vi "write wav file.vi"() -> ()   [LabVIEW 2018]
panel:
  in  "#Channels":i32=1
  in  "Device":u32
  in  "Resolution (bits)":i32=16
  in  "Sample rate (Hz)":dbl=44100.0
  in  "Path for Audio 1":path
  out "path out for Audio 1":path
  in  "Path for Audio 2":path
  out "Waveform Graph":dynamicdata(graph)
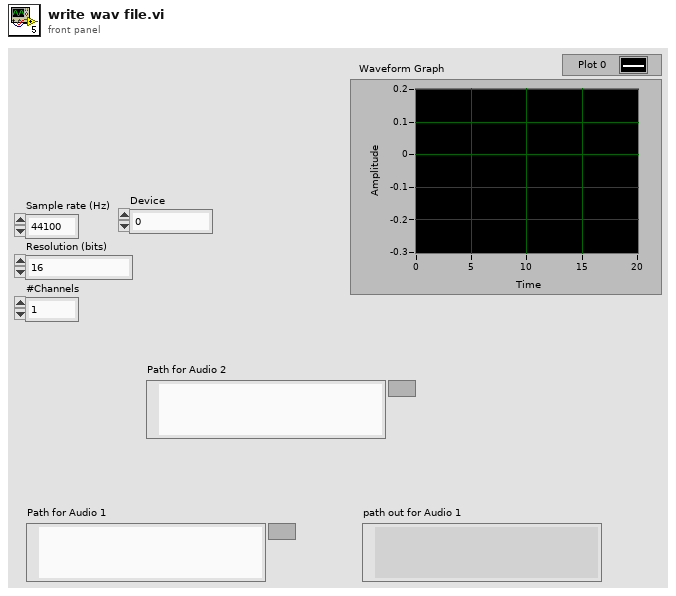
[diagram p1: front panel]
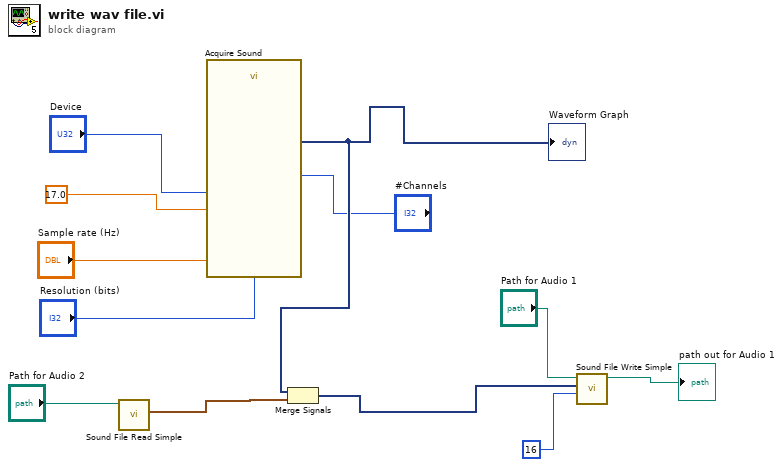
[diagram p0: block diagram]
diagram:
  n1 = call <vilib>:"Sound File Read Simple.vi"("path"="Path for Audio 2") -> ("data"=w11:waveform(dbl)[])  [unwired: 7 in, 3 out]
  n2 = call "Acquire Sound"("Device"="Device", "Duration (s)"=17.0, "Sample rate (Hz)"="Sample rate (Hz)", "#Channels"="#Channels", "Resolution (bits)"="Resolution (bits)") -> ("Data"=w12:dynamicdata)  [unwired: 13 in, 1 out]
  "Waveform Graph" <- w12
  n3 = Merge Signals(w12, w11) -> (w6:dynamicdata)
  n4 = call <vilib>:"Sound File Write Simple.vi"("bits per sample"=16, "data"=w6, "path"="Path for Audio 1") -> ("path out"=→"path out for Audio 1":path)  [unwired: 7 in, 1 out]
